vi "loadDataNodeBegin.vi"(8 "error in (no error)":errorcluster, 10 "XML Refnum in":refnum<file>, 11 "Parameters in":refnum<class "Parameters.lvclass">) -> (0 "error out":errorcluster, 2 "XML Refnum out":refnum<file>, 3 "Parameters out":refnum<class "Parameters.lvclass">)   [LabVIEW 2013, in "Parameters.lvclass"]
doc: "Part of the file loading process. Occurs at the beginning of a node being loaded. Loads the common xceDataNode data name and description."
uses:
  Parameters.lvclass
  xCE/xceDataNode/xceDataNode.lvclass
  xCE/xceNode/xceNode.lvclass
  XML Parser/XML Parser.lvclass
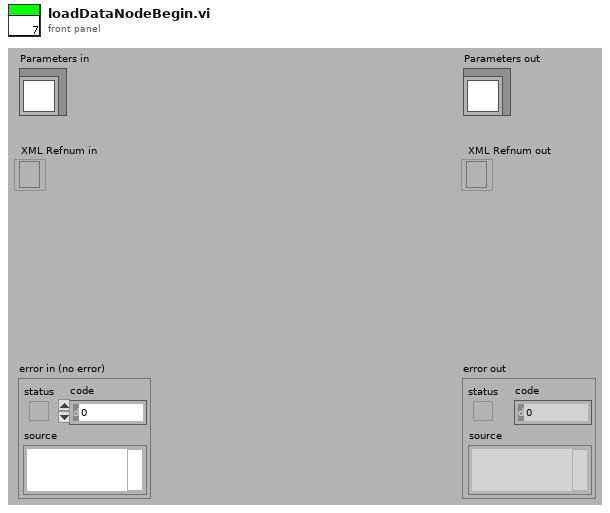
[diagram p1: front panel]
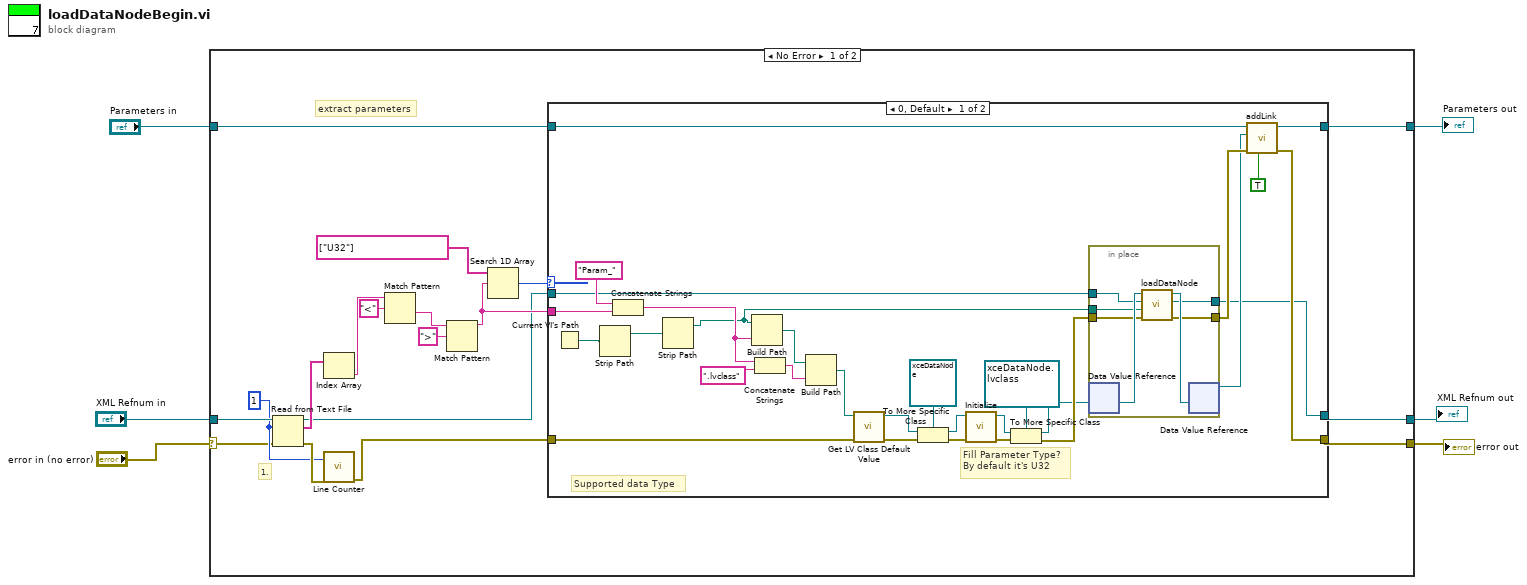
[diagram p0: block diagram]
diagram:
  n1 = case shown="No Error" "error in (no error)" {
    selector: "error in (no error)" -> [w7 w66]
    tunnel: [w24 w66] -> w2
    tunnel: [w23 w65] -> w1
    tunnel: "Parameters in" -> [w12 w65]
    tunnel: "XML Refnum in" -> [w11 w64]
    tunnel: [w22 w64] -> w3
    frame No Error {
      w8 = 1 ("count")
      # "extract parameters"
      # "1."
      n2 = Read from Text File(file (use dialog)=w11, count=w8, error in=w7) -> (refnum out=w13:refnum<file>, text=w15:string[], error out=w10:errorcluster)  [unwired: 1 in, 1 out]
      n3 = Index Array(array=w15) -> (element=w14:string)  [unwired: 1 in]
      n4 = call "Line Counter.vi"("error in (no error)"=w10, "# of lines to increment (1)"=w8) -> ("error out"=w9:errorcluster)  [unwired: 8 in, 1 out]
      n5 = Match Pattern(string=w14, regular expression="<") -> (after substring=w20:string)  [unwired: 1 in, 3 out]
      n6 = Match Pattern(string=w20, regular expression=">") -> (before substring=w16:string)  [unwired: 1 in, 3 out]
      n7 = Search 1D Array(1D array=string[] ["U32"] ("Allowed subNode[]"), element=w16) -> (index of element=w17:i32)  [unwired: 1 in]
      n8 = case shown="0, Default" w17 {
        tunnel: w12 -> [w29 w63]
        tunnel: w16 -> [w53 _]
        tunnel: w9 -> [w30 w61]
        tunnel: [w28 w63] -> w23
        tunnel: [w27 w61] -> w24
        tunnel: w13 -> [w26 w62]
        tunnel: [w25 w62] -> w22
        frame 0, Default {
          # "Fill Parameter Type?\nBy default it's U32"
          # "Supported data Type"
          n9 = Current VI's Path() -> (path=w51:path)
          n10 = Strip Path(path=w51) -> (stripped path=w50:path)  [unwired: 1 out]
          n11 = Concatenate Strings("Param_" ("string"), w53) -> (w32:string)
          n12 = Strip Path(path=w50) -> (stripped path=w31:path)  [unwired: 1 out]
          n13 = Build Path(base path=w31, name or relative path=w32) -> (appended path=w45:path)
          n14 = Concatenate Strings(w32, ".lvclass" ("string")) -> (w38:string)
          n15 = Build Path(base path=w45, name or relative path=w38) -> (appended path=w37:path)
          n16 = call <vilib>:"Get LV Class Default Value.vi"("error in (no error)"=w30, "class path"=w37) -> ("error out"=w34:errorcluster, "object"=w36:refnum<class>)  [unwired: 8 in]
          n17 = To More Specific Class(target class=refnum<class "xceDataNode.lvclass"> refnum ("xceDataNode.lvclass"), reference=w36, error in=w34) -> (specific class reference=w35:refnum<class "xceDataNode.lvclass">, error out=w33:errorcluster)
          n18 = call-dynamic "Initialize.vi"("error in"=w33, "xceDataNode in"=w35) -> ("error out"=w40:errorcluster, "Node*"=w41:refnum<data-value>)  [unwired: 8 in]
          n19 = To More Specific Class(target class=refnum<data-value> refnum ("data value reference"), reference=w41, error in=w40) -> (specific class reference=w44:refnum<data-value>, error out=w46:errorcluster)
          n20 = in-place {
            in-place-border: w31 -> [w59]
            in-place-border: w26 -> [w58]
            in-place-border: [w56] -> w25
            in-place-border: w46 -> [w55]
            in-place-border: [w54] -> w48
            n21 = in-place-dvr #1(w44) -> (w60:refnum<class "xceDataNode.lvclass">)  [unwired: 1 out]
            n22 = call "loadDataNode.vi"("error in (no error)"=w55, "CnfgEditorDir"=w59, "XML Refnum in"=w58, "xceDataNode in"=w60) -> ("error out"=w54:errorcluster, "XML Refnum out"=w56:refnum<file>, "xceDataNode out"=w57:refnum<class "xceDataNode.lvclass">)  [unwired: 5 in]
            n23 = in-place-dvr #1(w57) -> (w47:refnum<data-value>)  [unwired: 1 out]
          }
          n24 = call "addLink.vi"("Append to End"=TRUE, "error in (no error)"=w48, "subNode in"=w47, "superNode in"=w29) -> ("error out"=w27:errorcluster, "superNode out"=w28:refnum<class "Parameters.lvclass">)  [unwired: 5 in, 1 out]
        }
        frame 1 {
        }
      }
    }
    frame Error {
    }
  }
  "error out" <- w2
  "Parameters out" <- w1
  "XML Refnum out" <- w3
